vi "controlFixOutputVoltage.vi"(7 "set":bool, 8 "error in":errorcluster, 9 "Fixed Output Voltage in mV":i32, 10 "axis in":u8, 11 "connection ID":refnum<k5>) -> (0 "error out":errorcluster, 1 "Fixed Output Voltage in mV out":i32, 2 "axis out":u8, 3 "connection ID":refnum<k5>)   [LabVIEW 2016]
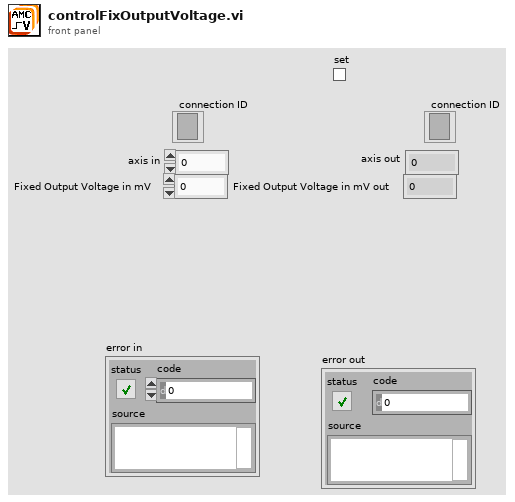
[diagram p1: front panel]
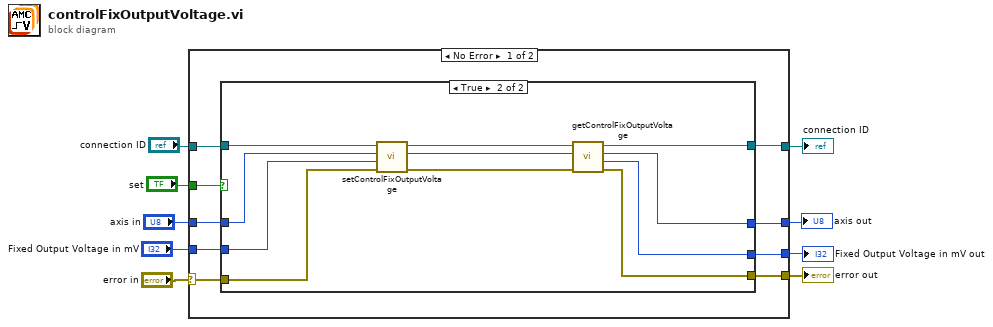
[diagram p0: block diagram]
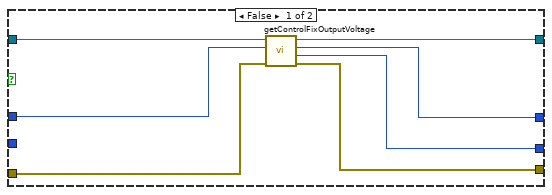
[diagram p2: hidden frame]
diagram:
  n1 = case shown="No Error" "error in" {
    selector: "error in" -> [w10 w40]
    tunnel: "axis in" -> [w17 w38]
    tunnel: [w11 w40] -> w8
    tunnel: [w13 w38] -> w7
    tunnel: "Fixed Output Voltage in mV" -> [w16 w39]
    tunnel: [w12 w39] -> w5
    tunnel: "set" -> [w18 _]
    tunnel: [w14 w37] -> w3
    tunnel: "connection ID" -> [w15 w37]
    frame No Error {
      n2 = case shown="True" w18 {
        tunnel: [w24 w26] -> w14
        tunnel: w15 -> [w25 w36]
        tunnel: w17 -> [w19 w34]
        tunnel: [w20 w27] -> w13
        tunnel: [w21 w28] -> w12
        tunnel: [w22 w29] -> w11
        tunnel: w16 -> [_ w33]
        tunnel: w10 -> [w23 w35]
        frame False {
          n3 = call "getControlFixOutputVoltage.vi"("error in"=w23, "axis"=w19, "connection ID"=w25) -> ("error out"=w22:errorcluster, "amplitude_mv"=w21:i32, "axis_out"=w20:i32, "connection ID"=w24:refnum<k5>)  [unwired: 5 in]
        }
        frame True {
          n4 = call "setControlFixOutputVoltage.vi"("error in"=w35, "amplitude_mv"=w33, "axis"=w34, "connection ID"=w36) -> ("error out"=w30:errorcluster, "axis_out"=w31:i32, "connection ID"=w32:refnum<k5>)  [unwired: 5 in]
          n5 = call "getControlFixOutputVoltage.vi"("error in"=w30, "axis"=w31, "connection ID"=w32) -> ("error out"=w29:errorcluster, "amplitude_mv"=w28:i32, "axis_out"=w27:i32, "connection ID"=w26:refnum<k5>)  [unwired: 5 in]
        }
      }
    }
    frame Error {
    }
  }
  "error out" <- w8
  "axis out" <- w7
  "Fixed Output Voltage in mV out" <- w5
  "connection ID" <- w3
